vi "main.vi"() -> ()   [LabVIEW 2020]
uses:
  <vilib>/Utility/NIReport.llb/Report Type.ctl
  <vilib>/addons/_office/excel.llb/Excel Get Data ([str]).vi
  <vilib>/Utility/NIReport.llb/NI_report.lvclass
  <vilib>/Utility/NIReport.llb/Excel/NI_Excel.lvclass
  <vilib>/addons/_office/NI_ReportGenerationToolkit.lvlib
  <vilib>/Utility/NIReport.llb/NI_ReportGenerationCore.lvlib
panel:
  in  "保存":bool
  in  "Item":T1={"OHM"=TRUE, "DCV"=TRUE, "ACV"=TRUE, "DCI"=TRUE, "ACI"=TRUE}
  out "文件名组":path[](array[path])
  in  "型号":u16(ring) items=["34401A"]
  in  "多功能源地址":refnum<visa-resource-name>
  in  "停止":bool
  in  "测量":bool
  in  "数表地址":refnum<visa-resource-name>
  in  "连接仪器":bool
  # "数字多用表自动化校准程序"
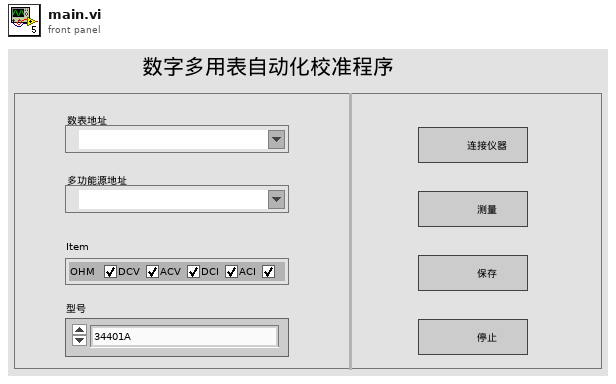
[diagram p1: front panel]
types:
  T1 = cluster{"OHM":bool, "DCV":bool, "ACV":bool, "DCI":bool, "ACI":bool}
  T2 = typedef "NI_ReportGenerationCore.lvlib/Report Type.ctl" = enum16{"HTML", "Word", "Excel"}
  T3 = enum16{"maximized", "minimized", "normal", "no change"}
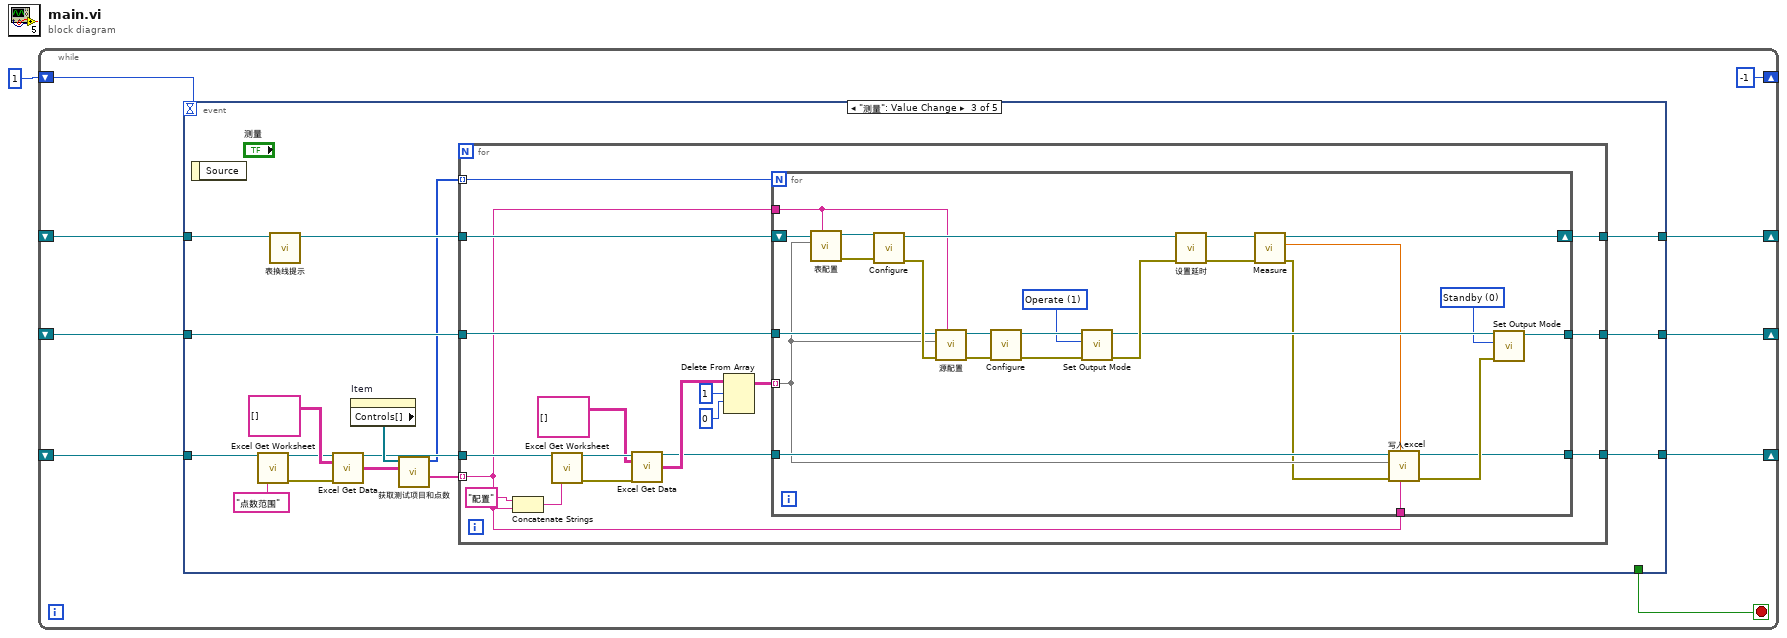
[diagram p0: block diagram]
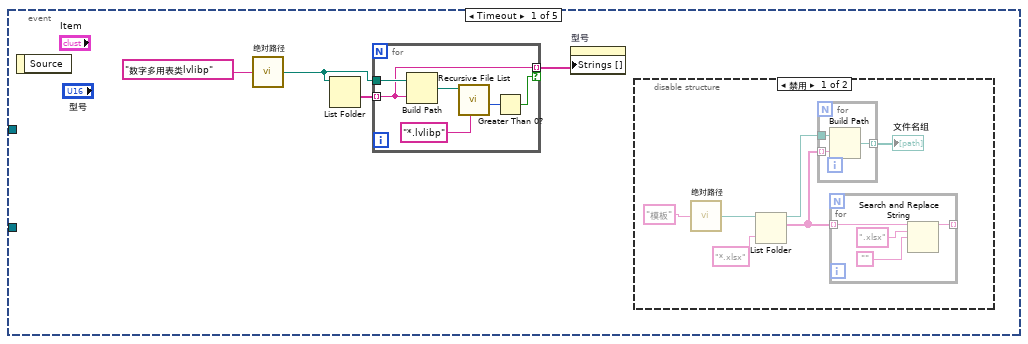
[diagram p2: hidden frame]
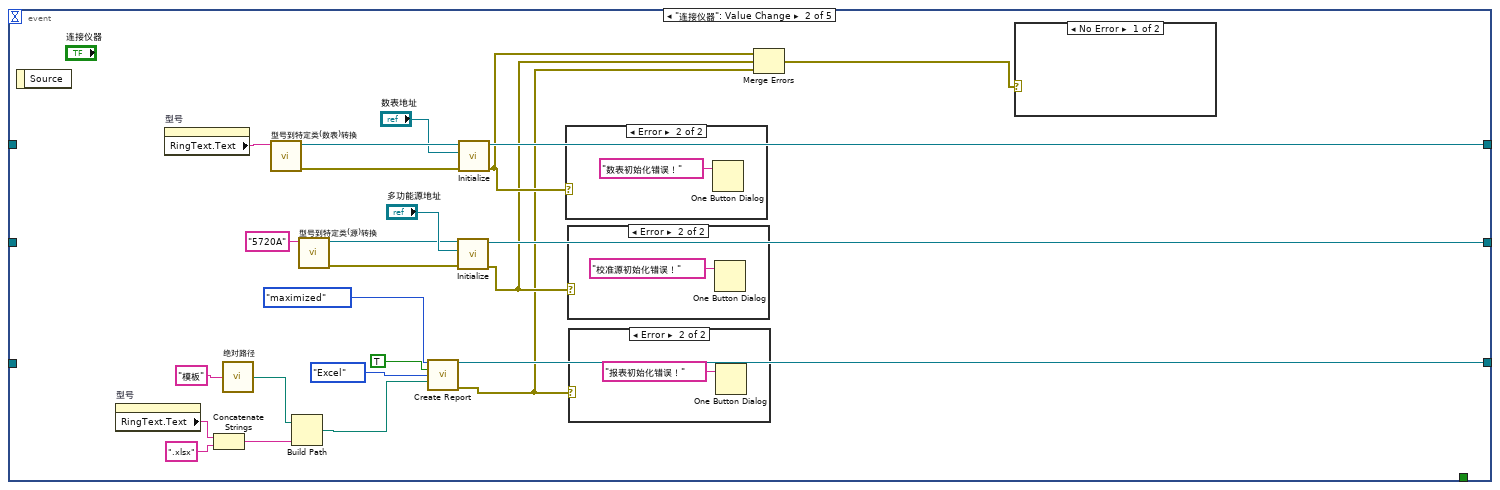
[diagram p4: hidden frame]
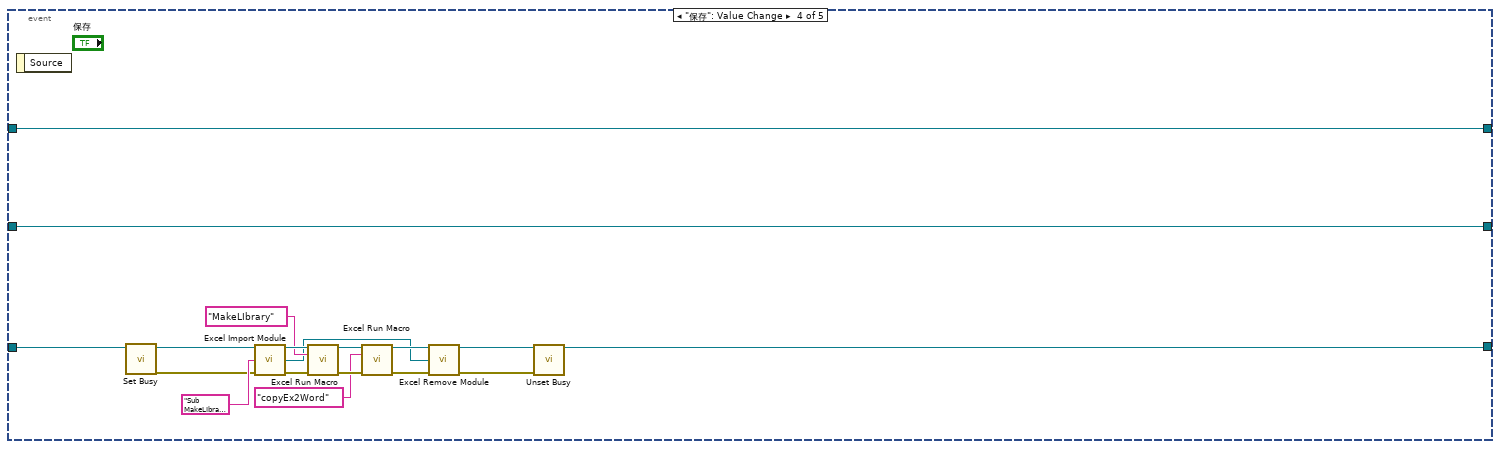
[diagram p9: hidden frame]
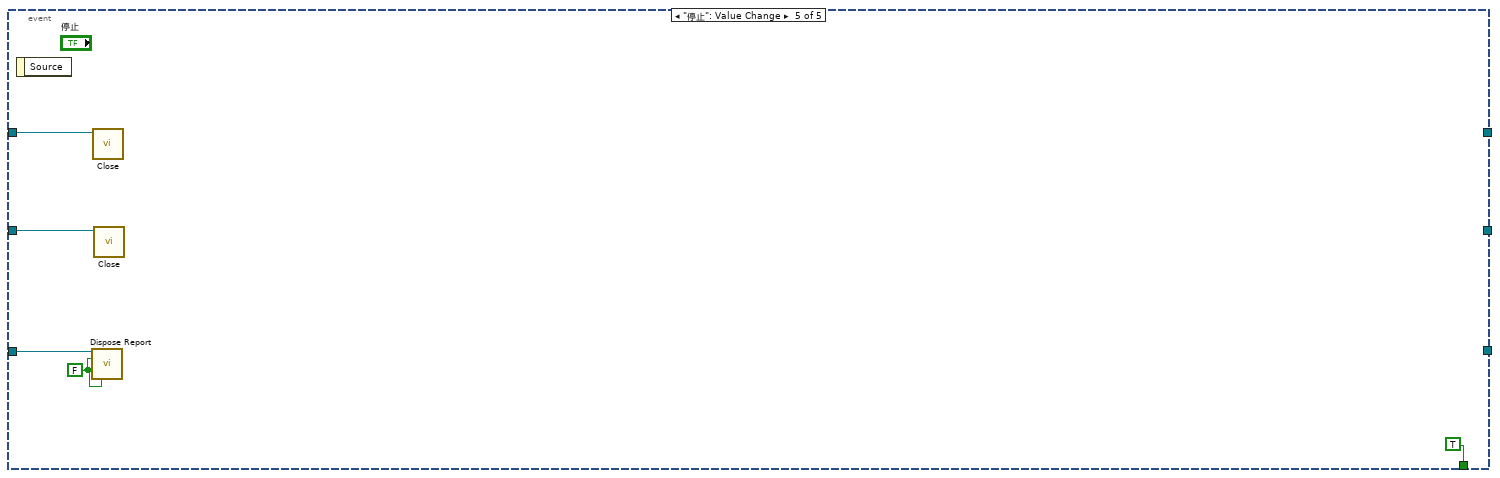
[diagram p10: hidden frame]
diagram:
  n1 = while {
    shift-right: [w9] -> _
    shift-left: _ -> [w7]
    shift-right: [w8] -> _
    shift-left: _ -> [w6]
    shift-right: [-1] -> _
    shift-left: 1 -> [w5]
    shift-right: [w3] -> _
    shift-left: _ -> [w2]
    stop <- w10 stop-if-true
    n2 = event shown="[2] \"测量\": Value Change" {
      selector: _ -> [_ _ _ _ _]
      dyn-events: _ -> [_ _ _ _ _]
      timeout: w5 -> [_ _ _ _ _]
      tunnel: [_ _ _ _ TRUE] -> w10
      tunnel: [_ w57 w75 w136 _] -> w9
      tunnel: [_ w56 w76 w135 _] -> w8
      tunnel: w7 -> [_ _ w73 w136 w140]
      tunnel: w6 -> [_ _ w74 w135 w139]
      tunnel: [_ w52 w61 w123 _] -> w3
      tunnel: w2 -> [_ _ w68 w134 w138]
      event Timeout {
        n3 = event-data() -> ()  [unwired: 1 in, 1 out]
        n4 = call "绝对路径.vi"("相对路径"="数字多用表类lvlibp" ("名称或相对路径")) -> ("绝对路径"=w12:path)
        n5 = List Folder(path=w12) -> (folder names=w14:string[])  [unwired: 3 in, 3 out]
        n6 = for {
          tunnel: w12 -> [w33]
          tunnel: w14 -> [w30] mode=indexing
          tunnel: [w30] -> w11 mode=indexing if=w29
          n7 = Build Path(base path=w33, name or relative path=w30) -> (appended path=w32:path)
          n8 = call <vilib>:"Recursive File List.vi"("pattern"="*.lvlibp", "Folder Path"=w32) -> ("Number of Files"=w31:i32)  [unwired: 5 in, 4 out]
          n9 = Greater Than 0?(x=w31) -> (x > 0?=w29:bool)
        }
        n10 = property on="型号" class="Ring (strict)"("Strings []"=w11) -> ()  [unwired: 2 in, 2 out]
        n11 = disable-structure shown="禁用" {
          frame Disabled {
            n12 = call "绝对路径.vi"("相对路径"="模板") -> ("绝对路径"=w18:path)
            n13 = List Folder(path=w18, pattern="*.xlsx" ("模式")) -> (path out=w17:path, filenames=w15:string[])  [unwired: 2 in, 2 out]
            n14 = for {
              tunnel: w17 -> [w27]
              tunnel: w15 -> [w26] mode=indexing
              tunnel: [w25] -> w16 mode=indexing
              n15 = Build Path(base path=w27, name or relative path=w26) -> (appended path=w25:path)
            }
            "文件名组" <- w16
            n16 = for {
              tunnel: w15 -> [w24] mode=indexing
              tunnel: [w21] -> _ mode=indexing
              n17 = Search and Replace String(input string=w24, search string=".xlsx" ("模式"), replace string="") -> (result string=w21:string)  [unwired: 5 in, 3 out]
            }
          }
          frame Enabled {
          }
        }
      }
      event "连接仪器": Value Change {
        n18 = event-data() -> ()  [unwired: 1 in, 1 out]
        n19 = property on="型号" class="Ring (strict)"() -> ("RingText.Text"=w46:string)  [unwired: 2 in, 2 out]
        n20 = property on="型号" class="Ring (strict)"() -> ("RingText.Text"=w41:string)  [unwired: 2 in, 2 out]
        n21 = Concatenate Strings(w46, ".xlsx" ("模式")) -> (w43:string)
        n22 = call "绝对路径.vi"("相对路径"="模板") -> ("绝对路径"=w44:path)
        n23 = call "型号到特定类(数表)转换.vi"("型号"=w41) -> ("错误输出"=w38:errorcluster, "DMM"=w40:refnum<class "数字多用表接口.lvclass">)  [unwired: 9 in]
        n24 = Build Path(base path=w44, name or relative path=w43) -> (appended path=w42:path)
        n25 = call "型号到特定类(源)转换.vi"("型号"="5720A") -> ("错误输出"=w35:errorcluster, "MC"=w37:refnum<class "多功能校准源接口.lvclass">)  [unwired: 9 in]
        n26 = call <vilib>:"Create Report.vi"("window state (normal)"=T3."maximized", "display alerts? (F)"=TRUE, "report type"=Report_Type."Excel", "template (empty)"=w42) -> ("report out"=w52:refnum<class "NI_report.lvclass">, "error out"=w49:errorcluster)  [unwired: 10 in]
        n27 = call-dynamic "Initialize.vi"("error in (no error)"=w35, "多功能源VISA"="多功能源地址", "多功能校准源接口 输入"=w37) -> ("error out"=w50:errorcluster, "多功能校准源接口 输出"=w56:refnum<class "多功能校准源接口.lvclass">)  [unwired: 7 in]
        n28 = call-dynamic "Initialize.vi"("error in (no error)"=w38, "VISA资源名称"="数表地址", "数字多用表接口 输入"=w40) -> ("error out"=w51:errorcluster, "数字多用表接口 输出"=w57:refnum<class "数字多用表接口.lvclass">)  [unwired: 7 in]
        n29 = case shown="Error" w51 {
          frame No Error {
          }
          frame Error {
            n30 = One Button Dialog(message="数表初始化错误！" ("消息")) -> ()  [unwired: 1 in, 1 out]
          }
        }
        n31 = case shown="Error" w50 {
          frame No Error {
          }
          frame Error {
            n32 = One Button Dialog(message="校准源初始化错误！" ("消息")) -> ()  [unwired: 1 in, 1 out]
          }
        }
        n33 = case shown="Error" w49 {
          frame No Error {
          }
          frame Error {
            n34 = One Button Dialog(message="报表初始化错误！" ("消息")) -> ()  [unwired: 1 in, 1 out]
          }
        }
        n35 = Merge Errors(w51, w50, w49) -> (w48:errorcluster)
        n36 = case shown="No Error" w48 {
          frame No Error {
          }
          frame Error {
          }
        }
      }
      event "测量": Value Change {
        n37 = event-data() -> ()  [unwired: 1 in, 1 out]
        n38 = call <vilib>:"Excel Get Worksheet.vi"("report in"=w68, "name (\"\")"="点数范围" ("name (\"\")")) -> ("report out"=w69:refnum<class "NI_report.lvclass">, "error out"=w70:errorcluster)  [unwired: 12 in]
        n39 = call-dynamic "表换线提示.vi"("数字多用表接口 输入"=w73) -> ("数字多用表接口 输出"=w72:refnum<class "数字多用表接口.lvclass">)  [unwired: 9 in, 1 out]
        n40 = call-poly <vilib>:"Excel Get Data.vi"("report in"=w69, "data type"=string[][] [], "error in (no error)"=w70) -> ("report out"=w63:refnum<class "NI_report.lvclass">, "data"=w65:string[][])  [unwired: 10 in, 1 out]
        n41 = property on="Item" class="Clust (strict)"() -> ("Controls[]"=w66:refnum<vi>[])  [unwired: 2 in, 2 out]
        n42 = call "获取测试项目和点数.vi"("Item&Count1"=w65, "Item"=w66) -> ("测量项目"=w64:string[], "测量点数"=w62:i32[])  [unwired: 8 in]
        n43 = for {
          tunnel: [w92] -> w76
          tunnel: w74 -> [w91]
          tunnel: w72 -> [w93]
          tunnel: [w94] -> w75
          tunnel: w64 -> [w78] mode=indexing
          tunnel: w63 -> [w90]
          tunnel: w62 -> [w80] mode=indexing
          tunnel: [w77] -> w61
          n44 = Concatenate Strings("配置", w78) -> (w81:string)
          n45 = call <vilib>:"Excel Get Worksheet.vi"("report in"=w90, "name (\"\")"=w81) -> ("report out"=w89:refnum<class "NI_report.lvclass">, "error out"=w88:errorcluster)  [unwired: 12 in]
          n46 = call-poly <vilib>:"Excel Get Data.vi"("report in"=w89, "data type"=string[][] [], "error in (no error)"=w88) -> ("report out"=w79:refnum<class "NI_report.lvclass">, "data"=w84:string[][])  [unwired: 10 in, 1 out]
          n47 = Delete From Array(array=w84, length=1 ("长度"), index (row)=0 ("长度")) -> (array with subset deleted=w83:string[][])  [unwired: 1 in, 1 out]
          n48 = for {
            N: w80 -> [_]
            tunnel: [w112] -> w92
            tunnel: w91 -> [w103]
            shift-right: [w120] -> w94
            shift-left: w93 -> [w107]
            tunnel: w83 -> [w100] mode=indexing
            tunnel: w78 -> [w104]
            tunnel: w79 -> [w101]
            tunnel: w78 -> [w99]
            tunnel: [w95] -> w77
            w111 = u32 0 items=["Standby", "Operate"] ("Output Mode")
            w115 = u32 1 items=["Standby", "Operate"] ("Output Mode")
            n49 = call "表配置.vi"("Item"=w104, "Arguments"=w100, "数字多用表接口输入"=w107) -> ("error out"=w109:errorcluster, "数字多用表接口输出"=w108:refnum<class "数字多用表接口.lvclass">)  [unwired: 7 in]
            n50 = call-dynamic "Configure.vi"("error in (no error)"=w109, "数字多用表接口 输入"=w108) -> ("error out"=w105:errorcluster, "数字多用表接口 输出"=w118:refnum<class "数字多用表接口.lvclass">)  [unwired: 8 in]
            n51 = call "源配置.vi"("Item"=w104, "error in (no error)"=w105, "Arguments"=w100, "多功能校准源接口输入"=w103) -> ("error out"=w106:errorcluster, "多功能校准源接口输出"=w102:refnum<class "多功能校准源接口.lvclass">)  [unwired: 6 in]
            n52 = call-dynamic "Configure.vi"("error in (no error)"=w106, "多功能校准源接口 输入"=w102) -> ("error out"=w110:errorcluster, "多功能校准源接口 输出"=w119:refnum<class "多功能校准源接口.lvclass">)  [unwired: 8 in]
            n53 = call-dynamic "Set Output Mode.vi"("error in (no error)"=w110, "Output Mode"=w115, "多功能校准源接口 输入"=w119) -> ("error out"=w116:errorcluster, "多功能校准源接口 输出"=w113:refnum<class "多功能校准源接口.lvclass">)  [unwired: 7 in]
            n54 = call-dynamic "设置延时.vi"("error in (no error)"=w116, "数字多用表接口 输入"=w118) -> ("error out"=w114:errorcluster, "数字多用表接口 输出"=w117:refnum<class "数字多用表接口.lvclass">)  [unwired: 8 in]
            n55 = call-dynamic "Measure.vi"("error in (no error)"=w114, "数字多用表接口 输入"=w117) -> ("error out"=w97:errorcluster, "Measurement"=w98:dbl, "数字多用表接口 输出"=w120:refnum<class "数字多用表接口.lvclass">)  [unwired: 7 in]
            n56 = call "写入excel.vi"("Item"=w99, "Measurement"=w98, "error in (no error)"=w97, "Arguments"=w100, "NI_report输入"=w101) -> ("error out"=w96:errorcluster, "report out"=w95:refnum<class "NI_report.lvclass">)  [unwired: 5 in]
            n57 = call-dynamic "Set Output Mode.vi"("error in (no error)"=w96, "Output Mode"=w111, "多功能校准源接口 输入"=w113) -> ("多功能校准源接口 输出"=w112:refnum<class "多功能校准源接口.lvclass">)  [unwired: 7 in, 1 out]
          }
        }
      }
      event "保存": Value Change {
        n58 = event-data() -> ()  [unwired: 1 in, 1 out]
        n59 = call <vilib>:"Set Busy.vi"() -> ("error out"=w122:errorcluster)  [unwired: 10 in, 1 out]
        n60 = call <vilib>:"Excel Import Module.vi"("report in"=w134, "module code (\"\")"="Sub MakeLIbrary()\n    ThisWorkbook.VBProject.References.AddFromguid \"{00020905-0000-0000-C000-000000000046}\", 8, 5\nEnd Sub\nSub copyEx2Word()\n    Dim appWD As Word.Application\n    Dim myDoc As Object\n    Dim myPath, docName, myItem, myScope, startItem, endItem As String\n    Dim cmWidth As Single\n    \n    Set appWD = CreateObject(\"word.Application\")\n    appWD.Visible = True\n    Set appWD = GetObject(, \"word.Application\")\n    myPath = Sheets(\"点数范围\").Range(\"B1\")\n    Set myDoc = GetObject(myPath)\n    appWD.Visible = True\n    startItem = Sheets(\"点数范围\").Range(\"B2\")\n    endItem = Sheets(\"点数范围\").Range(\"C2\")\n    cmWidth = Sheets(\"点数范围\").Range(\"B3\")\n    \n    For i = startItem To endItem\n        myItem = Sheets(\"点数范围\").Range(\"A\" & i)\n        myScope = Sheets(\"点数范围\").Range(\"D\" & i)\n        Sheets(myItem).Select\n        Range(myScope).Select\n        Selection.Copy\n        appWD.Selection.PasteSpecial Link:=False, DataType:=wdPasteOLEObject, Placement _\n            :=wdInLine, DisplayAsIcon:=False\n        Set e_shape = appWD.Selection.Document.InlineShapes(i - startItem + 1)\n        aHeight = e_shape.Height\n        aWidth = e_shape.Width\n        With e_shape\n            .LockAspectRatio = msoFalse\n            .Width = CentimetersToPoints(cmWidth) '1cm = 28.6磅\n            .Height = CentimetersToPoints(cmWidth * aHeight / aWidth)\n        End With\n    Next\n    'Application.CutCopyMode = False\n    Set appWD = Nothing\nEnd Sub\n\n\n" ("macro name"), "error in (no error)"=w122) -> ("report out"=w131:refnum<class "NI_report.lvclass">, "module reference"=w124:refnum<k7>, "error out"=w132:errorcluster)  [unwired: 10 in]
        n61 = call <vilib>:"Excel Run Macro.vi"("report in"=w131, "macro name"="MakeLIbrary", "error in (no error)"=w132) -> ("report out"=w129:refnum<class "NI_report.lvclass">, "error out"=w130:errorcluster)  [unwired: 10 in, 1 out]
        n62 = call <vilib>:"Excel Run Macro.vi"("report in"=w129, "macro name"="copyEx2Word", "error in (no error)"=w130) -> ("report out"=w125:refnum<class "NI_report.lvclass">, "error out"=w126:errorcluster)  [unwired: 10 in, 1 out]
        n63 = call <vilib>:"Excel Remove Module.vi"("report in"=w125, "module reference"=w124, "error in (no error)"=w126) -> ("report out"=w123:refnum<class "NI_report.lvclass">, "error out"=w121:errorcluster)  [unwired: 11 in]
        n64 = call <vilib>:"Unset Busy.vi"("error in (no error)"=w121) -> ()  [unwired: 10 in, 1 out]
      }
      event "停止": Value Change {
        w137 = FALSE ("save changes? (F)")
        n65 = event-data() -> ()  [unwired: 1 in, 1 out]
        n66 = call-dynamic "Dispose Report.vi"("report in"=w138, "wait until printing completed? (T)"=w137, "save changes? (F)"=w137, "close report? (T)"=w137) -> ()  [unwired: 11 in, 1 out]
        n67 = call-dynamic "Close.vi"("数字多用表接口 输入"=w140) -> ()  [unwired: 9 in, 2 out]
        n68 = call-dynamic "Close.vi"("多功能校准源接口 输入"=w139) -> ()  [unwired: 9 in, 2 out]
      }
    }
  }
